vi "Calculate Trigger Time (Falling Edge).vi"(8 "error in":errorcluster, 11 "Waveform In":waveform(dbl)) -> (0 "error out":errorcluster, 1 "Trigger Index (Samples)":dbl format="%#_2g", 2 "Trigger Time (Seconds)":dbl, 3 "Waveform Out":waveform(dbl))   [LabVIEW 2021]
doc: "Determine the time when the signal falls below the trigger value (2.5 volts)"
uses:
  <vilib>/measure/mamon.llb/Trigger Detection for 1 Channel.vi
  <vilib>/measure/NI_MAPro.lvlib
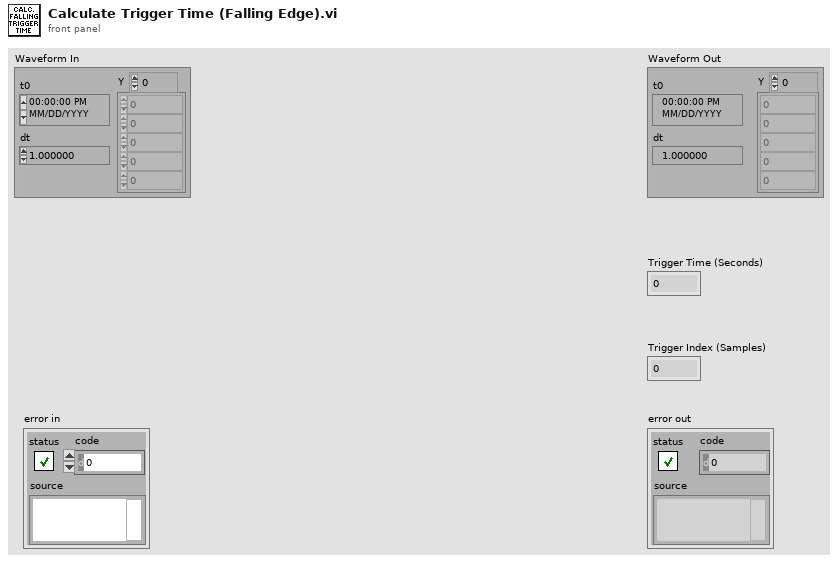
[diagram p1: front panel]
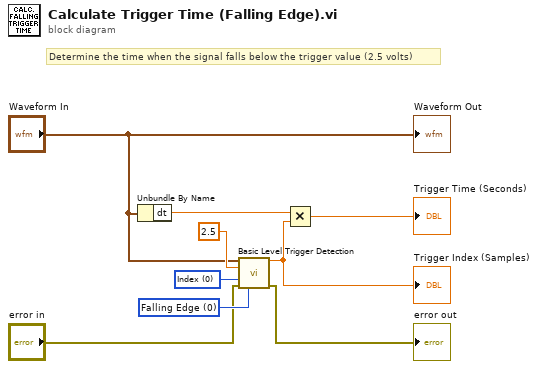
[diagram p0: block diagram]
diagram:
  w9 = u16 0 items=["Falling Edge", "Rising Edge"] ("trigger slope")
  w8 = u16 0 items=["Index", "Time"] ("location mode")
  # "Determine the time when the signal falls below the trigger value (2.5 volts)"
  n1 = Unbundle By Name("Waveform In") -> ("dt"=w5:dbl)
  n2 = call-poly <vilib>:"Basic Level Trigger Detection.vi"("signal in"="Waveform In", "level"=2.5, "location mode"=w8, "error in (no error)"="error in", "trigger slope"=w9) -> ("trigger location"=w4:dbl, "error out"=→"error out":errorcluster)  [unwired: 8 in, 1 out]
  "Trigger Index (Samples)" <- w4
  n3 = Multiply(x=w5, y=w4) -> (x*y=→"Trigger Time (Seconds)":dbl)
  "Waveform Out" <- "Waveform In"
